vi "stringTOnumber.vi"() -> ()   [LabVIEW 2019]
panel:
  out "1":dbl
  out "10":dbl
  out "100":dbl
  out "number":i32
  in  "stop":bool
  in  "string":string
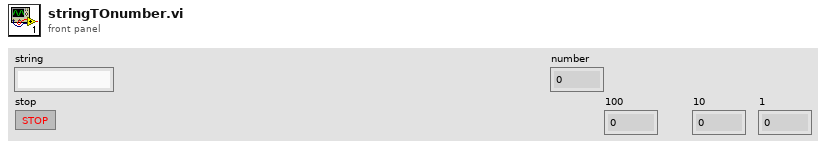
[diagram p1: front panel]
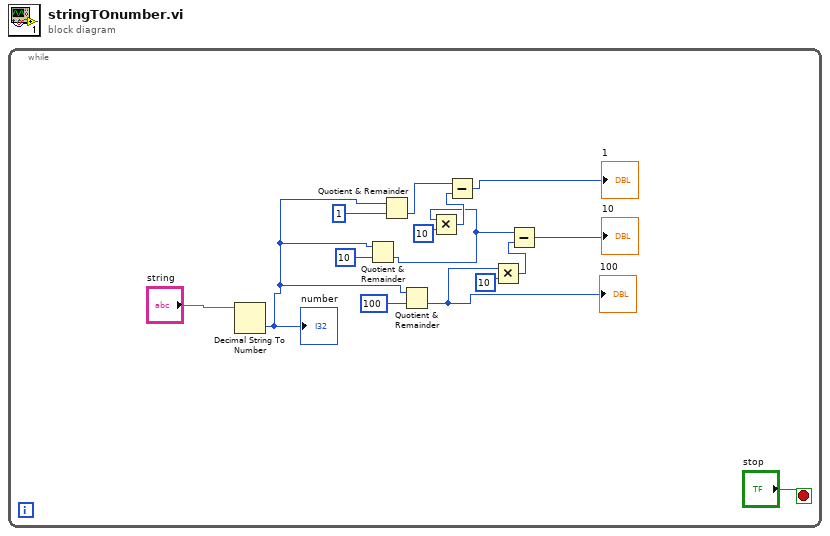
[diagram p0: block diagram]
diagram:
  n1 = while {
    stop <- "stop" stop-if-true
    n2 = Decimal String To Number(string="string") -> (number=w4:i32)  [unwired: 2 in, 1 out]
    "number" <- w4
    n3 = Quotient & Remainder(x=w4, y=10) -> (floor(x/y)=w1:i32)  [unwired: 1 out]
    n4 = Quotient & Remainder(x=w4, y=1) -> (floor(x/y)=w10:i32)  [unwired: 1 out]
    n5 = Quotient & Remainder(x=w4, y=100) -> (floor(x/y)=w2:i32)  [unwired: 1 out]
    "100" <- w2
    n6 = Multiply(x=w1, y=10) -> (x*y=w9:i32)
    n7 = Subtract(x=w10, y=w9) -> (x-y=→"1":i32)
    n8 = Multiply(x=w2, y=10) -> (x*y=w6:i32)
    n9 = Subtract(x=w1, y=w6) -> (x-y=→"10":i32)
  }
